vi "Run.vi"(9 "Team In":refnum<class "Team.lvclass">, 11 "MySquare in":refnum<class "MySquare.lvclass">) -> (1 "Team":refnum<class "Team.lvclass">, 2 "Run Result":T1={"Action"=enum."Move", "Direction"=enum."NW", "Replication"=refnum}, 3 "MySquare out":refnum<class "MySquare.lvclass">)   [LabVIEW 2020, in "SquareTeam.lvlib" / "MySquare.lvclass"]
doc: "This VI is called on every active square each turn of the game for the square to decide what action to take."
uses:
  MySquare.lvclass
  SquareBattle/Run Result.ctl
  SquareBattle/Square/Square.lvclass
  SquareBattle/Action.ctl
  SquareBattle/Direction.ctl
  SquareBattle/Team/Team.lvclass
  MyTeam/MyTeam.lvclass
  C:/dev/illuminatedg/sol-squarebattle/ProjectTemplates/Source/SummerOfLabVIEW/SquareBattle/template/SquareBattle/Team/Team.lvclass
  MySquare.lvclass/MySquare.ctl
  SquareBattle/SquareBattle.lvlib
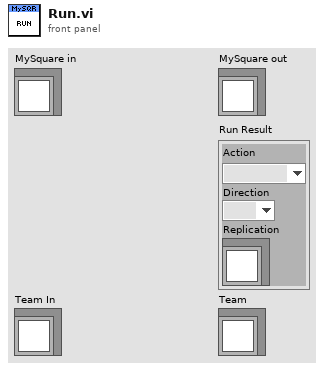
[diagram p1: front panel]
types:
  T1 = typedef "SquareBattle.lvlib/Run Result.ctl" = cluster{"Action":T2, "Direction":T3, "Replication":refnum<class "Square.lvclass">}
  T2 = typedef "SquareBattle.lvlib/Action.ctl" = enum16{"Wait", "Move", "Attack", "Replicate"}
  T3 = typedef "SquareBattle.lvlib/Direction.ctl" = enum16{"NW", "N", "NE", "E", "SE", "S", "SW", "W"}
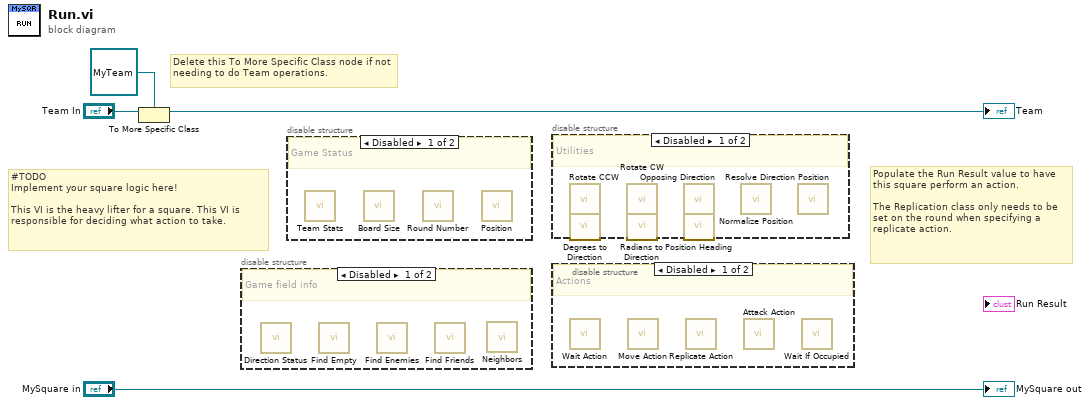
[diagram p0: block diagram]
diagram:
  # "Populate the Run Result value to have this square perform an action.\n\nThe Replication class only needs to be set on the round when specifying a replicate action."
  # "#TODO\nImplement your square logic here!\n\nThis VI is the heavy lifter for a square. This VI is responsible for deciding what action to take."
  # "Delete this To More Specific Class node if not needing to do Team operations."
  n1 = To More Specific Class(target class=refnum<class "MyTeam.lvclass"> refnum ("SquareTeam.lvlib:MyTeam.lvclass"), reference="Team In") -> (specific class reference=→"Team":refnum<class "MyTeam.lvclass">)  [unwired: 1 in, 1 out]
  n2 = disable-structure shown="Disabled" {
    frame Disabled {
      # "Game field info"
      n3 = call "Direction Status.vi"() -> ()  [unwired: 10 in, 2 out]
      n4 = call "Find Empty.vi"() -> ()  [unwired: 11 in, 1 out]
      n5 = call "Find Enemies.vi"() -> ()  [unwired: 11 in, 1 out]
      n6 = call "Find Friends.vi"() -> ()  [unwired: 11 in, 1 out]
      n7 = call "Neighbors.vi"() -> ()  [unwired: 11 in, 1 out]
    }
    frame Enabled {
    }
  }
  n8 = disable-structure shown="Disabled" {
    frame Disabled {
      # "Game Status"
      n9 = call "Team Stats.vi"() -> ()  [unwired: 11 in, 1 out]
      n10 = call "Board Size.vi"() -> ()  [unwired: 11 in, 1 out]
      n11 = call "Round Number.vi"() -> ()  [unwired: 11 in, 1 out]
      n12 = call "Position.vi"() -> ()  [unwired: 11 in, 1 out]
    }
    frame Enabled {
    }
  }
  n13 = disable-structure shown="Disabled" {
    frame Disabled {
      # "Utilities"
      n14 = call "Rotate CCW.vi"() -> ()  [unwired: 11 in, 1 out]
      n15 = call "Degrees to Direction.vi"() -> ()  [unwired: 11 in, 1 out]
      n16 = call "Rotate CW.vi"() -> ()  [unwired: 11 in, 1 out]
      n17 = call "Radians to Direction.vi"() -> ()  [unwired: 11 in, 1 out]
      n18 = call "Opposing Direction.vi"() -> ()  [unwired: 11 in, 1 out]
      n19 = call "Position Heading.vi"() -> ()  [unwired: 10 in, 2 out]
      n20 = call "Normalize Position.vi"() -> ()  [unwired: 10 in, 2 out]
      n21 = call "Resolve Direction Position.vi"() -> ()  [unwired: 9 in, 3 out]
    }
    frame Enabled {
    }
  }
  n22 = disable-structure shown="Disabled" {
    frame Disabled {
      # "Actions"
      n23 = call "Wait Action.vi"() -> ()  [unwired: 11 in, 1 out]
      n24 = call "Move Action.vi"() -> ()  [unwired: 11 in, 1 out]
      n25 = call "Replicate Action.vi"() -> ()  [unwired: 11 in, 1 out]
      n26 = call "Attack Action.vi"() -> ()  [unwired: 11 in, 1 out]
      n27 = call "Wait If Occupied.vi"() -> ()  [unwired: 11 in, 1 out]
    }
    frame Enabled {
    }
  }
  "MySquare out" <- "MySquare in"
